vi "DisposeDocument__slk_msxml.vi"(0 "document in":refnum<class "msxml document.lvclass">, 11 "error in (no error)":errorcluster) -> (15 "error out":errorcluster)   [LabVIEW 2020, in "MSXML.lvlib" / "msxml document.lvclass"]
doc: "Disposes MSXML Document object."
uses:
  msxml document.lvclass
  msxml document.lvclass/msxml document.ctl
panel:
  # "DisposeDocument__slk_msxml.vi\n\nDisposes MSXML Document object.\n\nNOTICE -- YOU MUST LEAVE THIS NOTICE IN PLACE.\n\nCopyright (c) 2004-2010 Shawn Liu <shawn.liu.cn@gmail.com>\n\nAll rights reserved."
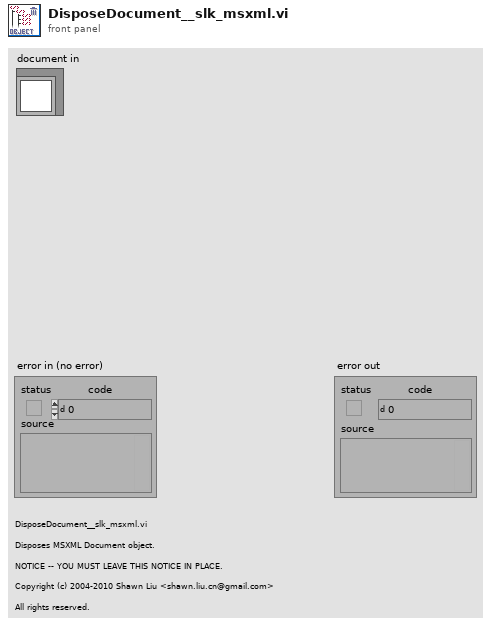
[diagram p1: front panel]
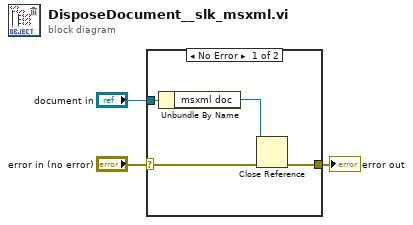
[diagram p0: block diagram]
diagram:
  n1 = case shown="No Error" "error in (no error)" {
    selector: "error in (no error)" -> [w5 w8]
    tunnel: [w6 w8] -> w1
    tunnel: "document in" -> [w7 _]
    frame No Error {
      n2 = Unbundle By Name(w7) -> ("msxml doc"=w4:refnum<k7>)
      n3 = Close Reference(reference=w4, error in (no error)=w5) -> (error out=w6:errorcluster)
    }
    frame Error {
    }
  }
  "error out" <- w1
